vi "LED Test.vi"(8 "error in (no error)":errorcluster, 9 "Lower LED Limit (V)":dbl=1.63, 10 "Upper LED Limit (V)":dbl=1.635, 11 "Meter":refnum<class "Meter.lvclass">) -> (0 "error out":errorcluster, 1 "Diode Voltage":dbl, 2 "LED Test Passed?":bool, 3 "Meter Out":refnum<class "Meter.lvclass">)   [LabVIEW 2010]
doc: "The LED on the DUT is tested by applying a current and measuring the voltage across the LED. This is accomplished by using the Diode Test function of the digital multimeter (DMM). If the resulting voltage is within the limits, the test is passed and a \"True\" is passed to the \"LED Test Passed?\" indicator. The LED Test VI also outputs the actual voltage that was measured."
uses:
  DSSP Modules/Input Classes/Meter/Meter.lvclass
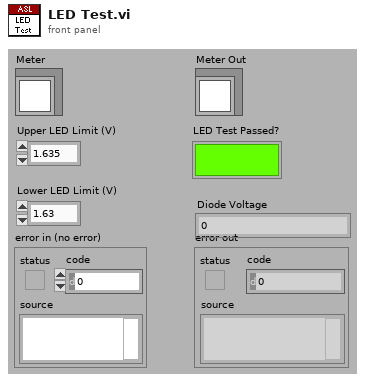
[diagram p1: front panel]
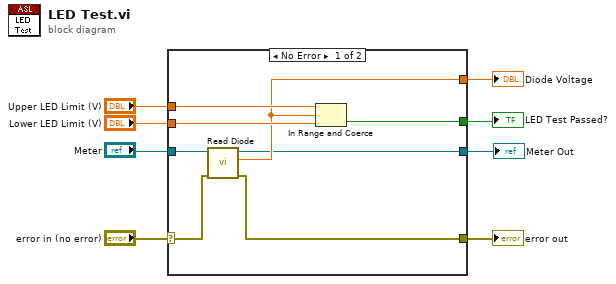
[diagram p0: block diagram]
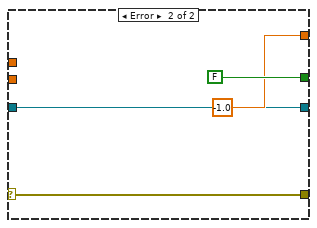
[diagram p2: hidden frame]
diagram:
  n1 = case shown="No Error" "error in (no error)" {
    selector: "error in (no error)" -> [w13 w20]
    tunnel: [w12 w20] -> w4
    tunnel: "Upper LED Limit (V)" -> [w16 _]
    tunnel: "Lower LED Limit (V)" -> [w15 _]
    tunnel: [w14 FALSE] -> w5
    tunnel: [w11 -1.0 ("Diode Voltage")] -> w3
    tunnel: "Meter" -> [w10 w17]
    tunnel: [w9 w17] -> w1
    frame No Error {
      n2 = call-dynamic "Read Diode.vi"("error in (no error)"=w13, "Meter In"=w10) -> ("error out"=w12:errorcluster, "Diode Voltage"=w11:dbl, "Meter Out"=w9:refnum<class "Meter.lvclass">)  [unwired: 7 out]
      n3 = In Range and Coerce(upper limit=w16, x=w11, lower limit=w15) -> (In Range?=w14:bool)  [unwired: 1 out]
    }
    frame Error {
    }
  }
  "LED Test Passed?" <- w5
  "error out" <- w4
  "Diode Voltage" <- w3
  "Meter Out" <- w1
